vi "Notch_Filter.vi"(11 "input data":fxp<+/-,16,1>) -> (3 "output data":fxp<+/-,16,3> format="%.14g")   [LabVIEW 2023]
doc: "----------------------\n\nThis filter is configured as follows:\n\n<b>Filter Configuration</b>\nType: Single Rate\nStructure: IIR Cascaded Second-Order Sections Form II Transposed\n\n<b>Input Data Type</b>\nType: fixed-point <±,16,1> [-1.000000E+0,9.999695E-1]:3.051758E-5\n\n<b>Output Data Type</b>\nType: fixed-point <±,16,3> [-4.000000E+0,3.999878E+0]:1.220703E-4\nRounding mode: Truncate\nOverflow mode: Wrap\n\n<b>Implementation</b>\nNumber of channels: 1\nMaximum input sampling rate per channel @ 40MHz: 8MHz\nGain processing: On Target\nMethod: Multiply-Accumulate\n\n<b>Execution Mode</b>\nOutside single-cycle Timed Loop\nThroughput: 5 cycles/call\n\n<b>Estimated Resources</b>\n2 32x32 multiplier"
uses:
  <vilib>/Platform/TimedLoop/XDataNode/timing_clust.ctl
  <vilib>/Platform/TimedLoop/XDataNode/nitl_modes.ctl
  <vilib>/Platform/TimedLoop/XDataNode/wakeup.ctl
  <vilib>/Platform/TimedLoop/XDataNode/XDataNode.xnode
  <vilib>/Platform/TimedLoop/XDataNode/XDNodeRunTimeDep.lvlib
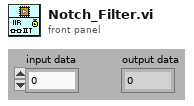
[diagram p1: front panel]
types:
  T1 = typedef "XDNodeRunTimeDep.lvlib/timing_clust.ctl" = cluster{"Expected End [f-1]":u64, "Actual End [f-1]":u64, "Finished Late? [f-1]":bool, "Expected End [i-1]":u64, "Actual End [i-1]":u64, "Finished Late? [i-1]":bool, "Expected Start [i]":u64, "Actual Start [i]":u64, "Expected Start [f]":u64, "Actual Start [f]":u64, "Source Name":string, "Structure Name":string, "Period":i64, "Deadline":i64, "Offset":i64, "Start":i64, "Priority":i32, "Timeout":i32, "Mode":T2, "Wakeup Reason":T3, "Error":errorcluster, "Source Type":string, "Secondary Source Type":string, "Global End Time":u64, "Global Start Time":u64, "Frame Duration":u64, "Iteration Duration":u64, "Assigned CPU":i32, "I/O Scan Engine Mode":u32}
  T2 = typedef "XDNodeRunTimeDep.lvlib/nitl_modes.ctl" = enum32{"No Change", "Process missed periods, maintain original phase", "Discard missed periods, maintain original phase", "Process missed periods, ignore original phase", "Discard missed periods, ignore original phase"}
  T3 = typedef "XDNodeRunTimeDep.lvlib/wakeup.ctl" = enum32{"Normal", "Aborted", "Asynchronous wakeup", "Timing source error", "Timed loop error", "Timeout"}
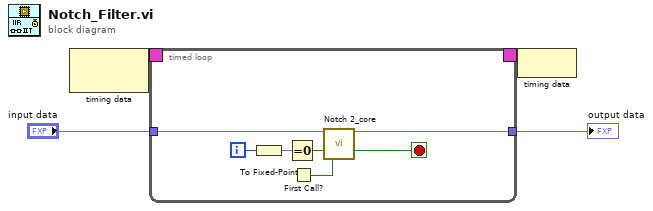
[diagram p0: block diagram]
diagram:
  n1 = node-c288() -> (w2:T1)  [unwired: 1 in]
  n2 = timed-loop "SCTL" {
    tunnel: "input data" -> [w6]
    tunnel: [w5] -> w3
    timing: w2 -> [_]
    timing-out: [_] -> w1
    i -> [w11]
    stop <- w7 stop-if-true
    n3 = To Fixed-Point(number=w11) -> (fixed-point=w10:fxp<+,12,12>)  [unwired: 1 out]
    n4 = Equal To 0?(x=w10) -> (x = 0?=w9:bool)
    n5 = First Call?() -> (First Call?: T/F=w8:bool)
    n6 = call "Notch 2_core"("input data"=w6, "input valid"=w9, "reset"=w8) -> ("output data"=w5:fxp<+/-,16,3>, "output valid"=w7:bool)  [unwired: 10 in, 1 out]
  }
  "output data" <- w3
  n7 = node-c288(w1) -> ()
